vi "Main Simulation.vi"() -> ()   [LabVIEW 2017]
uses:
  Calibrated Oculus Data.ctl
panel:
  out "Scene Display":refnum<vi>(3d-picture)
  out "error out":errorcluster
  in  "Boundary":T1={"X max"=310.0, "X min"=147.0, "Z max"=148.0, "Z min"=-92.0}
  in  "Freeze Head":bool
  out "Raw Oculus Data":T2
  out "Calibrated Oculus Data":T3
  in  "error in":errorcluster
  in  "Arm X Max":dbl=340.0
  in  "Arm X Min":dbl=90.0
  in  "VISA Refnum in":refnum<visa-resource-name>="ASRL3::INSTR"
  out "Calibration Complete":bool
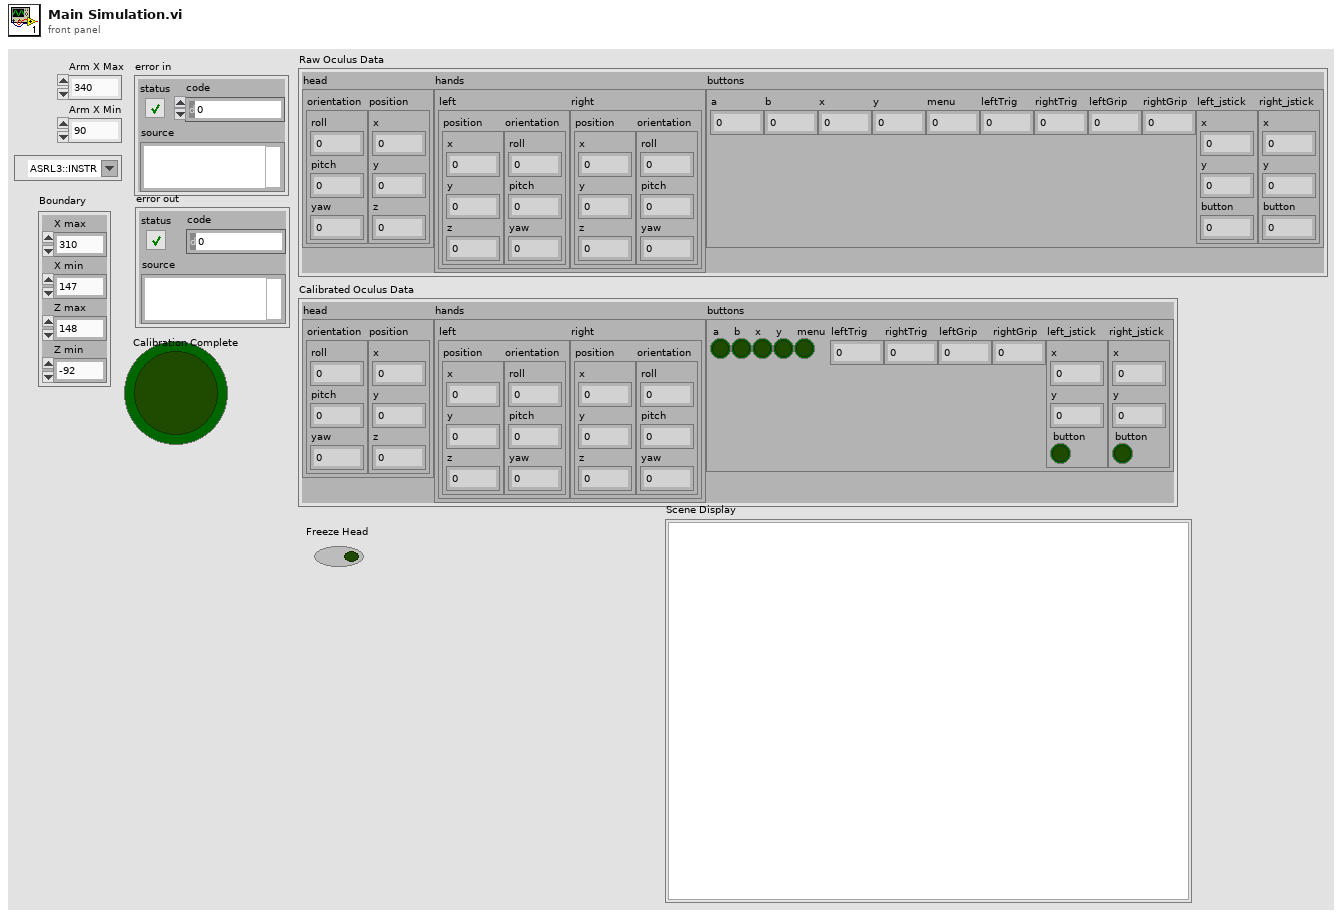
[diagram p1: front panel]
types:
  T1 = cluster{"X max":dbl, "X min":dbl, "Z max":dbl, "Z min":dbl}
  T2 = cluster{"head":cluster{"orientation":cluster{"roll":dbl, "pitch":dbl, "yaw":dbl}, "position":cluster{"x":dbl, "y":dbl, "z":dbl}}, "hands":cluster{"left":cluster{"position":cluster{"x":dbl, "y":dbl, "z":dbl}, "orientation":cluster{"roll":dbl, "pitch":dbl, "yaw":dbl}}, "right":cluster{"position":cluster{"x":dbl, "y":dbl, "z":dbl}, "orientation":cluster{"roll":dbl, "pitch":dbl, "yaw":dbl}}}, "buttons":cluster{"a":i32, "b":i32, "x":i32, "y":i32, "menu":i32, "leftTrig":dbl, "rightTrig":dbl, "leftGrip":dbl, "rightGrip":dbl, "left_jstick":cluster{"x":dbl, "y":dbl, "button":i32}, "right_jstick":cluster{"x":dbl, "y":dbl, "button":i32}}}
  T3 = typedef "Calibrated Oculus Data.ctl" = cluster{"head":cluster{"orientation":cluster{"roll":dbl, "pitch":dbl, "yaw":dbl}, "position":cluster{"x":dbl, "y":dbl, "z":dbl}}, "hands":cluster{"left":cluster{"position":cluster{"x":dbl, "y":dbl, "z":dbl}, "orientation":cluster{"roll":dbl, "pitch":dbl, "yaw":dbl}}, "right":cluster{"position":cluster{"x":dbl, "y":dbl, "z":dbl}, "orientation":cluster{"roll":dbl, "pitch":dbl, "yaw":dbl}}}, "buttons":cluster{"a":bool, "b":bool, "x":bool, "y":bool, "menu":bool, "leftTrig":dbl, "rightTrig":dbl, "leftGrip":dbl, "rightGrip":dbl, "left_jstick":cluster{"x":dbl, "y":dbl, "button":bool}, "right_jstick":cluster{"x":dbl, "y":dbl, "button":bool}}}
  T4 = cluster{"left":cluster{"Center":cluster{"x":dbl, "y":dbl, "z":dbl}, "Max":dbl}, "right":cluster{"Center":cluster{"x":dbl, "y":dbl, "z":dbl}, "Max":dbl}}
  T5 = cluster{"head":cluster{"orientation":cluster{"roll":dbl, "pitch":dbl, "yaw":dbl}, "position":cluster{"x":dbl, "y":dbl, "z":dbl}}, "hands":cluster{"left":cluster{"position":cluster{"x":dbl, "y":dbl, "z":dbl}, "orientation":cluster{"roll":dbl, "pitch":dbl, "yaw":dbl}}, "right":cluster{"position":cluster{"x":dbl, "y":dbl, "z":dbl}, "orientation":cluster{"roll":dbl, "pitch":dbl, "yaw":dbl}}}, "buttons":cluster{"a":bool, "b":bool, "x":bool, "y":bool, "menu":bool, "leftTrig":dbl, "rightTrig":dbl, "leftGrip":dbl, "rightGrip":dbl, "left_jstick":cluster{"x":dbl, "y":dbl, "button":bool}, "right_jstick":cluster{"x":dbl, "y":dbl, "button":bool}}}
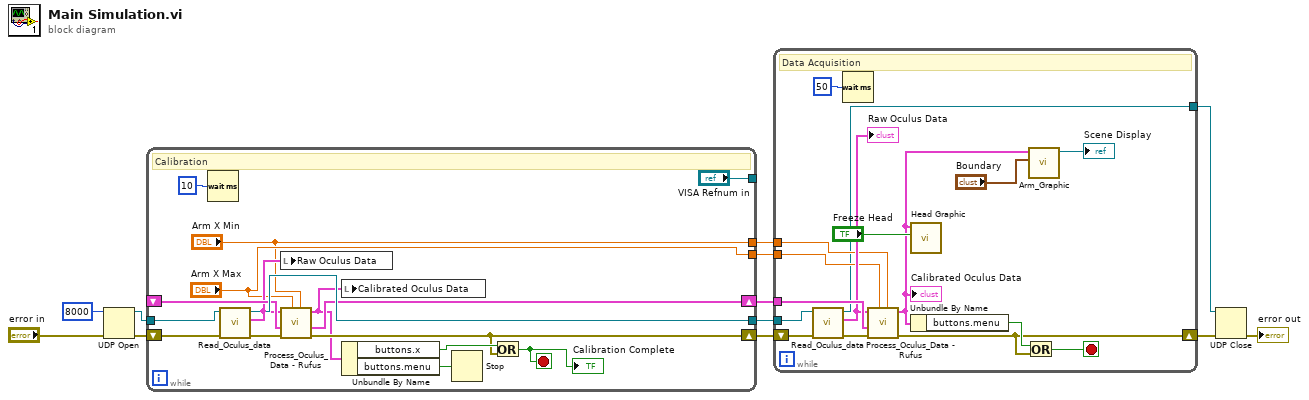
[diagram p0: block diagram]
diagram:
  n1 = UDP Open(8:"error in", 11:8000) -> (port=w10:refnum<k16>, 0:w11:errorcluster)  [unwired: 3 in, 1 out]
  n2 = while "Calibration" {
    tunnel: w10 -> [w27]
    tunnel: [w26] -> w7
    shift-right: [w20] -> w5
    shift-left: w11 -> [w28]
    tunnel: ["VISA Refnum in"] -> _
    shift-right: [w18] -> w6
    shift-left: _ -> [w19]
    tunnel: ["Arm X Max"] -> w4
    tunnel: ["Arm X Min"] -> w3
    stop <- w24 stop-if-true
    # "Calibration"
    n3 = Wait (ms)(milliseconds to wait=u32 10) -> ()  [unwired: 1 out]
    n4 = call "Read_Oculus_data.vi"("error in (no error)"=w28, "UDP Network Connection in"=w27) -> ("error out"=w21:errorcluster, "Cluster"=w17:T2, "UDP Network Connection out"=w26:refnum<k16>)  [unwired: 7 in]
    n5 = local write "Raw Oculus Data"(w17) -> ()
    n6 = call "Process_Oculus_Data - Rufus.vi"("Arm X Min"="Arm X Min", "Arm X Max"="Arm X Max", "error in"=w21, "Calibration Data in"=w19, "Oculus Data In"=w17) -> ("error out"=w20:errorcluster, "Calibration Data out"=w18:T4, "Oculus Data out"=w15:T5)  [unwired: 4 in]
    n7 = local write "Calibrated Oculus Data"(w15) -> ()
    n8 = Unbundle By Name(w15) -> ("buttons.x"=w22:bool, "buttons.menu"=w16:bool)
    n9 = Stop(stop? (T)=w16) -> ()
    n10 = Or(x=w22, y=w20) -> (x .or. y?=w24:bool)
    "Calibration Complete" <- w24
  }
  n11 = while "Data Aquisition" {
    shift-right: [w41] -> w8
    shift-left: w5 -> [w38]
    tunnel: w7 -> [w39]
    tunnel: w6 -> [w42]
    tunnel: w4 -> [w35]
    tunnel: w3 -> [w34]
    tunnel: [w32] -> w1
    stop <- w40 stop-if-true
    # "Data Acquisition"
    n12 = call "Read_Oculus_data.vi"("error in (no error)"=w38, "UDP Network Connection in"=w39) -> ("error out"=w37:errorcluster, "Cluster"=w36:T2, "UDP Network Connection out"=w32:refnum<k16>)  [unwired: 7 in]
    "Raw Oculus Data" <- w36
    n13 = Wait (ms)(milliseconds to wait=u32 50) -> ()  [unwired: 1 out]
    n14 = call "Process_Oculus_Data - Rufus.vi"("Arm X Min"=w34, "Arm X Max"=w35, "error in"=w37, "Calibration Data in"=w42, "Oculus Data In"=w36) -> ("error out"=w41:errorcluster, "Oculus Data out"=w31:T5)  [unwired: 4 in, 1 out]
    "Calibrated Oculus Data" <- w31
    n15 = call "Head Graphic.vi"("Stop"="Freeze Head", "Oculus Data in"=w31) -> ()  [unwired: 10 in]
    n16 = Unbundle By Name(w31) -> ("buttons.menu"=w43:bool)
    n17 = Or(x=w43, y=w41) -> (x .or. y?=w40:bool)
    n18 = call "Arm_Graphic.vi"("Boundary"="Boundary", "Calibrated Oculus Data"=w31) -> ("Scene Display"=→"Scene Display":refnum<vi>)  [unwired: 9 in]
  }
  n19 = UDP Close(connection ID=w1, 8:w8) -> (error out=→"error out":errorcluster)  [unwired: 1 out]
